vi "Merge Stream States.vi"(0 "request to restart":bool[](array[boolean]), 2 "reset":bool, 7 "ready for start in":bool[](array[boolean]), 9 "enable":bool[](array[boolean]), 11 "state in":T1[](array[typedef])) -> (4 "request to restart out":bool, 6 "ready to restart disable":bool, 8 "ready for start out":bool, 15 "state out":T1 caption="stream.state 0")   [LabVIEW 2018, in "GettingStarted_5774_FPGA.lvlib"]
uses:
  GettingStarted_5774_FPGA.lvlib
  <instrlib>/_niInstr/Streaming/v1/Common/Stream State.ctl
  <instrlib>/_niInstr/Streaming/v1/Common/niInstr Streaming v1 Common.lvlib
  <instrlib>/_niInstr/Basic Elements/v1/FPGA/niInstr Basic Elements v1 FPGA.lvlib
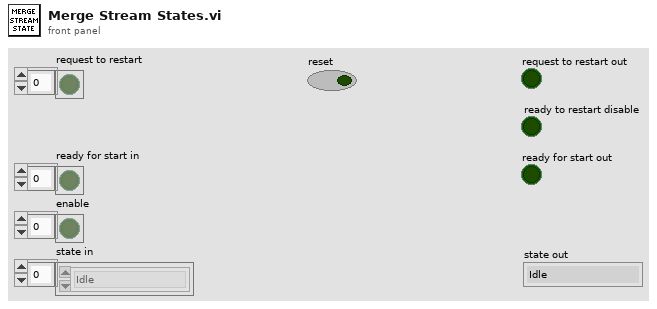
[diagram p1: front panel]
types:
  T1 = typedef "niInstr Streaming v1 Common.lvlib/Stream State.ctl" = enum8{"Idle", "Finite Transfer", "Continuous", "Done", "Error", "Not Ready", "Cancel"}
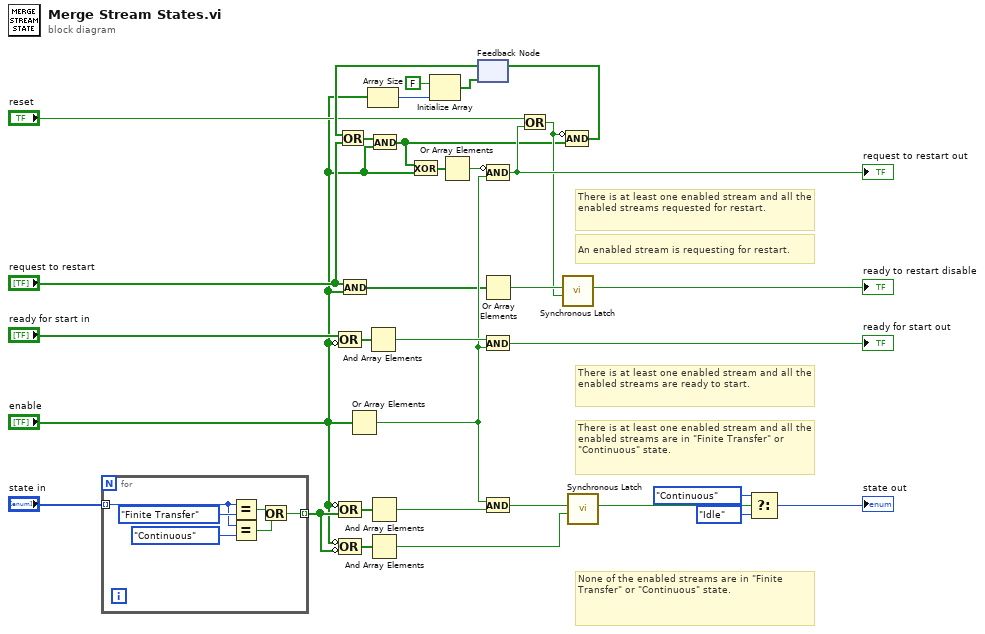
[diagram p0: block diagram]
diagram:
  # "An enabled stream is requesting for restart."
  # "There is at least one enabled stream and all the enabled streams requested for restart."
  # "None of the enabled streams are in \"Finite Transfer\" or \"Continuous\" state."
  # "There is at least one enabled stream and all the enabled streams are in \"Finite Transfer\" or \"Continuous\" state."
  # "There is at least one enabled stream and all the enabled streams are ready to start."
  n1 = for {
    tunnel: "state in" -> [w38] mode=indexing
    tunnel: [w34] -> w23 mode=indexing
    n2 = Equal?(x=w38, y=Stream_State."Finite Transfer") -> (x = y?=w36:bool)
    n3 = Equal?(x=w38, y=Stream_State."Continuous") -> (x = y?=w35:bool)
    n4 = Or(x=w36, y=w35) -> (x .or. y?=w34:bool)
  }
  n5 = Compound Arithmetic op=OR("ready for start in", invert "enable") -> (w33:bool[])
  n6 = Compound Arithmetic op=OR(invert "enable", w23) -> (w28:bool[])
  n7 = Compound Arithmetic op=OR(invert "enable", invert w23) -> (w22:bool[])
  n8 = And(x="request to restart", y="enable") -> (x .and. y?=w7:bool[])
  n9 = Or Array Elements(Boolean array="enable") -> (logical OR=w17:bool)
  n10 = Array Size(array="enable") -> (size(s)=w10:i32)
  n11 = And Array Elements(Boolean array=w33) -> (logical AND=w32:bool)
  n12 = And Array Elements(Boolean array=w28) -> (logical AND=w29:bool)
  n13 = And Array Elements(Boolean array=w22) -> (logical AND=w21:bool)
  n14 = Initialize Array(FALSE, w10) -> (w8:bool[])
  n15 = feedback #1(w8) -> (w19:bool[])
  n16 = Or(x=w19, y="request to restart") -> (x .or. y?=w6:bool[])
  n17 = And(x=w6, y="enable") -> (x .and. y?=w2:bool[])
  n18 = Exclusive Or(1:"enable", 2:w2) -> (0:w5:bool[])
  n19 = Or Array Elements(Boolean array=w5) -> (logical OR=w4:bool)
  n20 = Or Array Elements(Boolean array=w7) -> (logical OR=w15:bool)
  n21 = And(x=w32, y=w17) -> (x .and. y?=→"ready for start out":bool)
  n22 = And(x=w17, y=w29) -> (x .and. y?=w27:bool)
  n23 = Compound Arithmetic op=AND(invert w4, w17) -> (w16:bool)
  "request to restart out" <- w16
  n24 = Or(x="reset", y=w16) -> (x .or. y?=w14:bool)
  n25 = call <instrlib>:"Synchronous Latch.vi"("clear"=w14, "set"=w15) -> ("out"=→"ready to restart disable":bool)  [unwired: 9 in]
  n26 = Compound Arithmetic op=AND(invert w14, w2) -> (w13:bool[])
  n27 = feedback-in #1(w13) -> ()
  n28 = call <instrlib>:"Synchronous Latch.vi"("clear"=w21, "set"=w27) -> ("out"=w26:bool)  [unwired: 9 in]
  n29 = Select(t=Stream_State."Continuous" ("state"), s=w26, f=Stream_State."Idle" ("state")) -> (s? t:f=→"state out":T1)
